vi "GetPrice.vi"(8 "Error In":errorcluster, 11 "reference in":refnum<class "MenuItem.lvclass">) -> (0 "Error Out":errorcluster, 2 "Price":dbl, 3 "reference in":refnum<class "MenuItem.lvclass">)   [LabVIEW 2020, in "MenuItem.lvclass"]
uses:
  MenuItem.lvclass
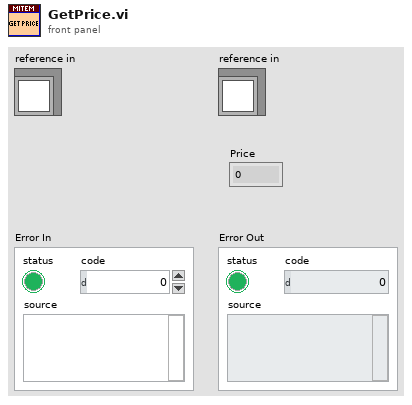
[diagram p1: front panel]
types:
  T1 = typedef "MenuItem.lvclass/ObjectAttributes.ctl" = cluster{"Name":string, "Description":string, "Price":dbl, "Vegetarian":bool}
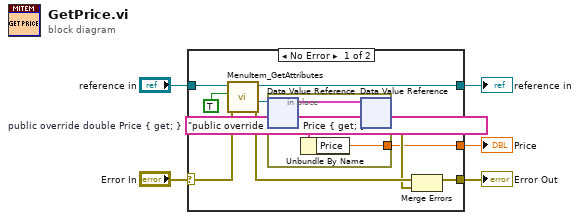
[diagram p0: block diagram]
diagram:
  (unwired) "public override double Price { get; }"  # public override double Price { get; }
  n1 = case shown="No Error" "Error In" {
    selector: "Error In" -> [w14 w18]
    tunnel: [w12 w18] -> w4
    tunnel: [w9 w17] -> w2
    tunnel: "reference in" -> [w10 w17]
    tunnel: [w6 _] -> w1
    frame No Error {
      n2 = call "MenuItem_GetAttributes.vi"("error in (no error)"=w14, "OnlyGetDvrReference(False)"=TRUE, "reference in"=w10) -> ("error out"=w13:errorcluster, "DataRef"=w8:refnum<data-value>, "reference out"=w9:refnum<class "MenuItem.lvclass">)  [unwired: 5 in, 1 out]
      n3 = in-place {
        in-place-border: [w16] -> w6
        n4 = in-place-dvr #1(w8) -> (w15:T1)  [unwired: 1 out]
        n5 = Unbundle By Name(w15) -> ("Price"=w16:dbl)
        n6 = in-place-dvr #1(w15) -> (w11:errorcluster)  [unwired: 1 out]
      }
      n7 = Merge Errors(w13, w11) -> (w12:errorcluster)
    }
    frame Error {
    }
  }
  "Error Out" <- w4
  "reference in" <- w2
  "Price" <- w1
